vi "file_int app.vi"() -> ()   [LabVIEW 2012, in "LightPipes.lvlib"]
uses:
  LightPipes.lvlib
panel:
  in  "Source Intensity":path=path "C:/Users/Green Beret/Documents/Visual Studio 2012/Projects/LightPipes/LightPipes/lp12src/LabView/images/original/initial.pgm"
  in  "Final Beam":path=path "C:/Users/Green Beret/Documents/Visual Studio 2012/Projects/LightPipes/LightPipes/lp12src/LabView/images/final_beam.pgm"
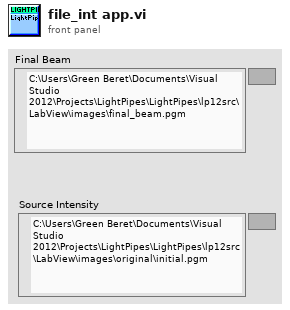
[diagram p1: front panel]
types:
  T1 = cluster{"n_grid":i32, "@dummy control@":i8, "@dummy control@":i8, "@dummy control@":i8, "@dummy control@":i8, "size":dbl, "lambda":dbl, "int1":i32, "int2":i32, "int3":i32, "@dummy control@":i8, "@dummy control@":i8, "@dummy control@":i8, "@dummy control@":i8, "double1":dbl, "double2":dbl, "double3":dbl, "real":u32, "imaginary":u32}
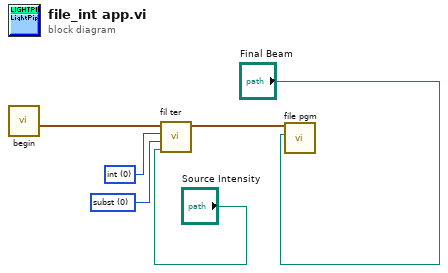
[diagram p0: block diagram]
diagram:
  w5 = i16 0 items=["subst", "mult"] ("multiplication/ substitution")
  w6 = i16 0 items=["int", "pha"] ("intensity / phase")
  n1 = call "begin.vi"() -> ("field out"=w4:T1)  [unwired: 11 in]
  n2 = call "fil ter.vi"("Path"="Source Intensity", "multiplication/ substitution"=w5, "intensity / phase"=w6, "field"=w4) -> ("field out"=w3:T1)  [unwired: 6 in, 1 out]
  n3 = call "file pgm.vi"("Path"="Final Beam", "field"=w3) -> ()  [unwired: 8 in, 2 out]
